vi "Psi from quaternions (SubVI).vi"(6 "Array in":dbl[](array[numeric]), 9 "Array 3":dbl[](array[numeric]), 10 "Array 4":dbl[](array[numeric]), 11 "Array 5":dbl[](array[numeric])) -> (3 "Array out":dbl[](array[numeric]))   [LabVIEW 2011]
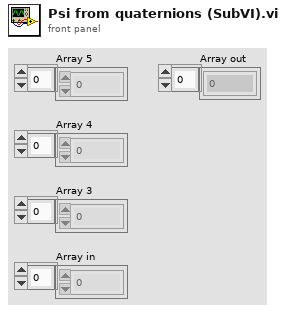
[diagram p1: front panel]
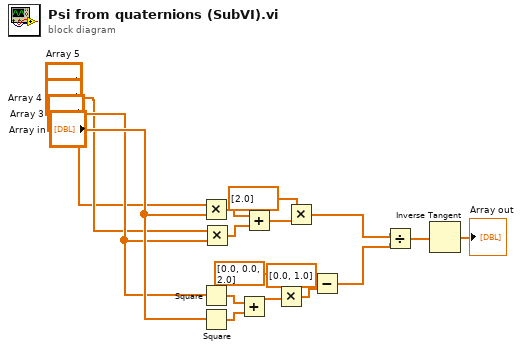
[diagram p0: block diagram]
diagram:
  n1 = Multiply(x="Array 5", y="Array in") -> (x*y=w8:dbl[])
  n2 = Square(x="Array 3") -> (x^2=w13:dbl[])
  n3 = Square(x="Array in") -> (x^2=w12:dbl[])
  n4 = Multiply(x="Array 4", y="Array 3") -> (x*y=w9:dbl[])
  n5 = Add(x=w13, y=w12) -> (x+y=w11:dbl[])
  n6 = Add(x=w8, y=w9) -> (x+y=w10:dbl[])
  n7 = Multiply(x=dbl[] [0.0, 0.0, 2.0], y=w11) -> (x*y=w7:dbl[])
  n8 = Multiply(x=dbl[] [2.0], y=w10) -> (x*y=w6:dbl[])
  n9 = Subtract(x=dbl[] [0.0, 1.0], y=w7) -> (x-y=w5:dbl[])
  n10 = Divide(x=w6, y=w5) -> (x/y=w1:dbl[])
  n11 = Inverse Tangent(1:w1) -> (0:→"Array out":dbl[])
